vi "waaca_main.vi"() -> ()   [LabVIEW 2016]
uses:
  <vilib>/ptbypt/NI_PtbyPt.lvlib
panel:
  out "Running average (3s)":dbl(graph)
  out "Running average (3s)":dbl format="%#.1f"
  out "Running average (3s)":dbl(knob) scale=0.0..100.0
  in  "SNAPSHOT":bool
  in  "TARE":bool
  in  "Stop":bool
  out "Tared average":dbl
  out "Pre-tare average":dbl
  out "AC kg mean":dbl
  out "BD kg mean":dbl
  out "BD Voltage mean":dbl format="%.3f"
  out "AC Voltage mean":dbl format="%.3f"
  out "DEBUG AC":dynamicdata(graph)
  out "DEBUG BD":dynamicdata(graph)
  out "DEBUG BOTH":dynamicdata(graph)
  # "===================================== DEBUGGING =========================================="
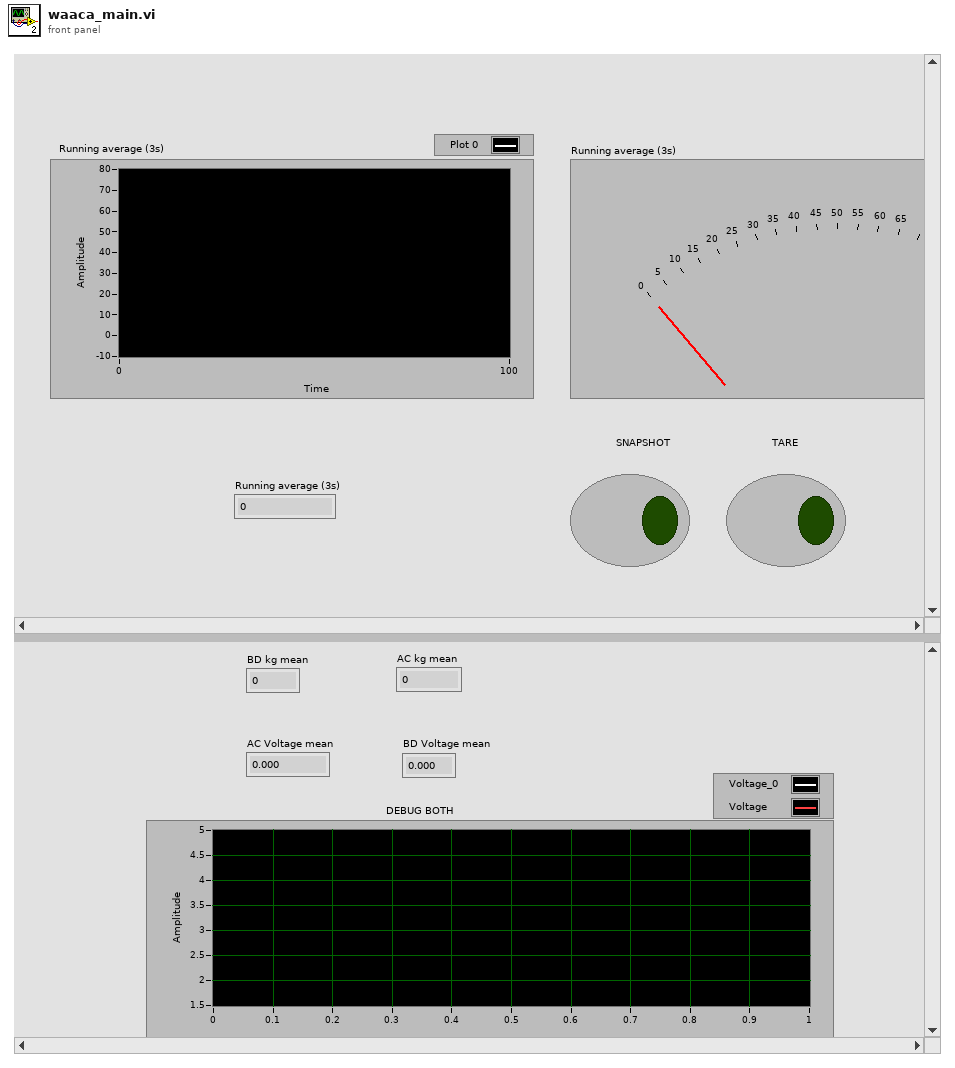
[diagram p1: front panel]
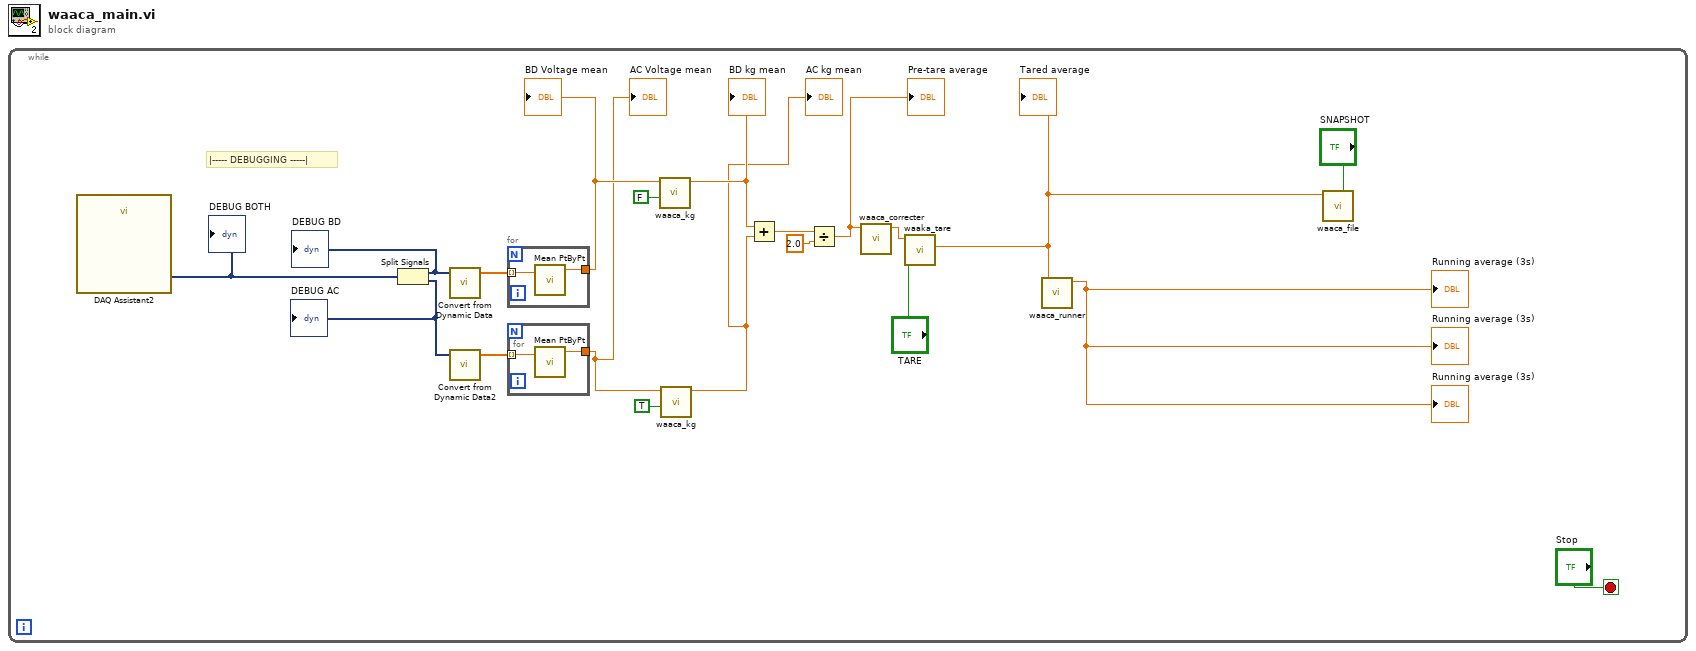
[diagram p0: block diagram]
diagram:
  n1 = while {
    stop <- "Stop" stop-if-true
    # "|----- DEBUGGING -----|"
    n2 = call "DAQ Assistant2"() -> ("data"=w12:dynamicdata)  [unwired: 17 in, 2 out]
    "DEBUG BOTH" <- w12
    n3 = Split Signals(w12) -> (w19:dynamicdata, w18:dynamicdata)  [unwired: 2 in]
    "DEBUG BD" <- w19
    "DEBUG AC" <- w18
    n4 = call "Convert from Dynamic Data"("Dynamic Data Type"=w19) -> ("Array"=w17:dbl[])  [unwired: 3 in]
    n5 = call "Convert from Dynamic Data2"("Dynamic Data Type"=w18) -> ("Array"=w16:dbl[])  [unwired: 3 in]
    n6 = for {
      tunnel: w17 -> [w22] mode=indexing
      tunnel: [w21] -> w10
      n7 = call <vilib>:"Mean PtByPt.vi"("x"=w22) -> ("mean"=w21:dbl)  [unwired: 3 in, 1 out]
    }
    "BD Voltage mean" <- w10
    n8 = for {
      tunnel: [w24] -> w3
      tunnel: w16 -> [w23] mode=indexing
      n9 = call <vilib>:"Mean PtByPt.vi"("x"=w23) -> ("mean"=w24:dbl)  [unwired: 3 in, 1 out]
    }
    "AC Voltage mean" <- w3
    n10 = call "waaca_kg.vi"("AC/BD"=FALSE, "Voltage in"=w10) -> ("KG output"=w8:dbl)  [unwired: 9 in]
    "BD kg mean" <- w8
    n11 = call "waaca_kg.vi"("AC/BD"=TRUE, "Voltage in"=w3) -> ("KG output"=w2:dbl)  [unwired: 9 in]
    "AC kg mean" <- w2
    n12 = Add(x=w8, y=w2) -> (x+y=w15:dbl)
    n13 = Divide(x=w15, y=2.0) -> (x/y=w5:dbl)
    "Pre-tare average" <- w5
    n14 = call "waaca_correcter.vi"("Input weight"=w5) -> ("Corrected output weight"=w4:dbl)  [unwired: 10 in]
    n15 = call "waaka_tare.vi"("Update"="TARE", "Input weight"=w4) -> ("Output weight"=w6:dbl)  [unwired: 9 in]
    "Tared average" <- w6
    n16 = call "waaca_runner.vi"("Numeric"=w6) -> ("Numeric 2"=→"Running average (3s)" →"Running average (3s)" →"Running average (3s)":dbl)  [unwired: 8 in]
    n17 = call "waaca_file.vi"("Boolean"="SNAPSHOT", "INPUT R.AVG"=w6) -> ()  [unwired: 10 in]
  }
